vi "Save File DOE Create Filename Sub.vi"(8 "Error In":errorcluster, 9 "Filepath":T1, 10 "LV Program":T9=enum."DOE Stand", 11 "Appliance Details":T3={"FileVersionInfo"={"FileVersion"="", "ProductName"="", "InternalName"="", "CompanyName"="", "LegalCopyright"="", "FileDescription"=""}, "Dishwasher Info"={"Open Cup Weight (gm):"=0.0, "Auto Cup Weight (gm):"=0.0, "Detergent-Dish:"="", "Inlet Temperature-Dish:"="", "Cycle Mode-Dish:"="", "Unit Control-Dish:"="", "Manufacturer-Dish:"=""}, "Washer Info"={"Hot Water Temperature (Fahrenheit):"="", "Cold Water Temperature (Fahrenheit):"="", "Capacity (cu.ft):"=0.0, "Initial Cloth Weight:"=0.0, "Cloth Lot:"=0, "Model Family:"="", "Program Name:"="", "Cycle Selection:"="", "Wash Temperature:"="", "Rinse Temperature:"="", "Load Size:"=""}, "File Name Output Array"=[], "Calibration Output Array"=[], "Appliance Common"={"Engineer:"="", "Model Number:"="", "Serial Number:"="", "Comments:"="", "Station ID:"="", "Technician:"="", "TR Number:"="", "Lab ID:"="", "Voltage:"="", "Water Pressure (PSI):"="", "Test Date:"="", "Computer Name:"="", "IP Address:"="", "Ambient RH:"="", "Frequency:"="", "Build:"="", "Filename:"="", "Test Type:"="", "Load Run #:"=0, "Ambient Temperature (F):"="", "File Path:"=path "", "Cycles Per Year"=60}, "Water Heater"={"Heating Mode:"=""}, "Dryer"={"Heat Setting:"="", "Washer Water Temperature (60 ± 5°F):"=60, "Water Hardness (PPM):"=17, "Dryness Setting:"="", "Dryer Type:"="", "Exhaust:"="", "Drying Cycle:"="", "Load Type:"="", "Nominal Load Weight"="", "Dryer Initial IMC Data"={"Measured IMC (lbs)"=7.0, "Actual Initial RMC (%)"=7.0, "RMC (Desired %)"=100.0, "Bone Dry Wt(lbs)"=7.0, "Tolerance(%)"=5.0, "Actual Final RMC (%)"=7.0, "CEF (lbf/kWh)"=0.0, "Minimum Weight (lbf)"=0.0, "Average Weight (lbf)"=0.0, "Maximum Weight (lbf)"=0.0, "Measured IMC In Range?"=FALSE, "Moisture Reduction Factor"=55.5, "Field Use Factor"=1.04, "Empty Dryer Cold Weigth"=0.0, "Energy Standard"=enum."D2-Automatic Dryer", "Weight Cloth (lbs)"=0.0, "Relative Moisture Content (%)"=0.0, "Relative Moisture Content - Avg (%)"=0.0}}} {"Dryer"."Dryer Initial IMC Data"."Maximum Weight (lbf)" format="%03_6g"; "Dryer"."Dryer Initial IMC Data"."Average Weight (lbf)" format="%03_6g"; "Dryer"."Dryer Initial IMC Data"."Minimum Weight (lbf)" format="%03_6g"; "Dryer"."Dryer Initial IMC Data"."CEF (lbf/kWh)" format="%03_6g"; "Dryer"."Dryer Initial IMC Data"."Actual Final RMC (%)" format="%03_6g"; "Dryer"."Dryer Initial IMC Data"."Tolerance(%)" format="%0#_6g"; "Dryer"."Dryer Initial IMC Data"."Bone Dry Wt(lbs)" format="%03_6g"; "Dryer"."Dryer Initial IMC Data"."RMC (Desired %)" format="%0#_6g"; "Dryer"."Dryer Initial IMC Data"."Actual Initial RMC (%)" format="%03_6g"; "Dryer"."Dryer Initial IMC Data"."Measured IMC (lbs)" format="%0#_6g"}) -> (0 "Error Out":errorcluster, 2 "Filepath Output":T1, 3 "Appliance Details Output":T3={"FileVersionInfo"={"FileVersion"="", "ProductName"="", "InternalName"="", "CompanyName"="", "LegalCopyright"="", "FileDescription"=""}, "Dishwasher Info"={"Open Cup Weight (gm):"=0.0, "Auto Cup Weight (gm):"=0.0, "Detergent-Dish:"="", "Inlet Temperature-Dish:"="", "Cycle Mode-Dish:"="", "Unit Control-Dish:"="", "Manufacturer-Dish:"=""}, "Washer Info"={"Hot Water Temperature (Fahrenheit):"="", "Cold Water Temperature (Fahrenheit):"="", "Capacity (cu.ft):"=0.0, "Initial Cloth Weight:"=0.0, "Cloth Lot:"=0, "Model Family:"="", "Program Name:"="", "Cycle Selection:"="", "Wash Temperature:"="", "Rinse Temperature:"="", "Load Size:"=""}, "File Name Output Array"=[], "Calibration Output Array"=[], "Appliance Common"={"Engineer:"="", "Model Number:"="", "Serial Number:"="", "Comments:"="", "Station ID:"="", "Technician:"="", "TR Number:"="", "Lab ID:"="", "Voltage:"="", "Water Pressure (PSI):"="", "Test Date:"="", "Computer Name:"="", "IP Address:"="", "Ambient RH:"="", "Frequency:"="", "Build:"="", "Filename:"="", "Test Type:"="", "Load Run #:"=0, "Ambient Temperature (F):"="", "File Path:"=path "", "Cycles Per Year"=60}, "Water Heater"={"Heating Mode:"=""}, "Dryer"={"Heat Setting:"="", "Washer Water Temperature (60 ± 5°F):"=60, "Water Hardness (PPM):"=17, "Dryness Setting:"="", "Dryer Type:"="", "Exhaust:"="", "Drying Cycle:"="", "Load Type:"="", "Nominal Load Weight"="", "Dryer Initial IMC Data"={"Measured IMC (lbs)"=7.0, "Actual Initial RMC (%)"=7.0, "RMC (Desired %)"=100.0, "Bone Dry Wt(lbs)"=7.0, "Tolerance(%)"=5.0, "Actual Final RMC (%)"=7.0, "CEF (lbf/kWh)"=0.0, "Minimum Weight (lbf)"=0.0, "Average Weight (lbf)"=0.0, "Maximum Weight (lbf)"=0.0, "Measured IMC In Range?"=FALSE, "Moisture Reduction Factor"=55.5, "Field Use Factor"=1.04, "Empty Dryer Cold Weigth"=0.0, "Energy Standard"=enum."D2-Automatic Dryer", "Weight Cloth (lbs)"=0.0, "Relative Moisture Content (%)"=0.0, "Relative Moisture Content - Avg (%)"=0.0}}} {"Dryer"."Dryer Initial IMC Data"."Maximum Weight (lbf)" format="%03_6g"; "Dryer"."Dryer Initial IMC Data"."Average Weight (lbf)" format="%03_6g"; "Dryer"."Dryer Initial IMC Data"."Minimum Weight (lbf)" format="%03_6g"; "Dryer"."Dryer Initial IMC Data"."CEF (lbf/kWh)" format="%03_6g"; "Dryer"."Dryer Initial IMC Data"."Actual Final RMC (%)" format="%03_6g"; "Dryer"."Dryer Initial IMC Data"."Tolerance(%)" format="%0#_6g"; "Dryer"."Dryer Initial IMC Data"."Bone Dry Wt(lbs)" format="%03_6g"; "Dryer"."Dryer Initial IMC Data"."RMC (Desired %)" format="%0#_6g"; "Dryer"."Dryer Initial IMC Data"."Actual Initial RMC (%)" format="%03_6g"; "Dryer"."Dryer Initial IMC Data"."Measured IMC (lbs)" format="%0#_6g"})   [LabVIEW 2016, in "File Setup.lvlib"]
uses:
  File Setup.lvlib
  Save File.lvlib
  File Setup (Public)/Type Definition/Save File DOE LabView Program.ctl
  File Setup (Public)/Type Definition/Save File DISH Dishwasher Details.ctl
  <vilib>/Platform/fileVersionInfo.llb/FileVersionInformation.ctl
  File Setup (Public)/Type Definition/Save File DOE Data Save Filepaths.ctl
  File Setup (Public)/Type Definition/Save File DOE File Path Control.ctl
  Custom Pallet Controls/Custom Pallet String.ctl
  File Setup (Public)/Type Definition/DPT IMC Data.ctl
  Washer DOE/Type Definitions/DOE Appliance Common.ctl
  Washer DOE/Type Definitions/DOE Dryer Standard.ctl
panel:
  in  "File Extension:":string="csv"
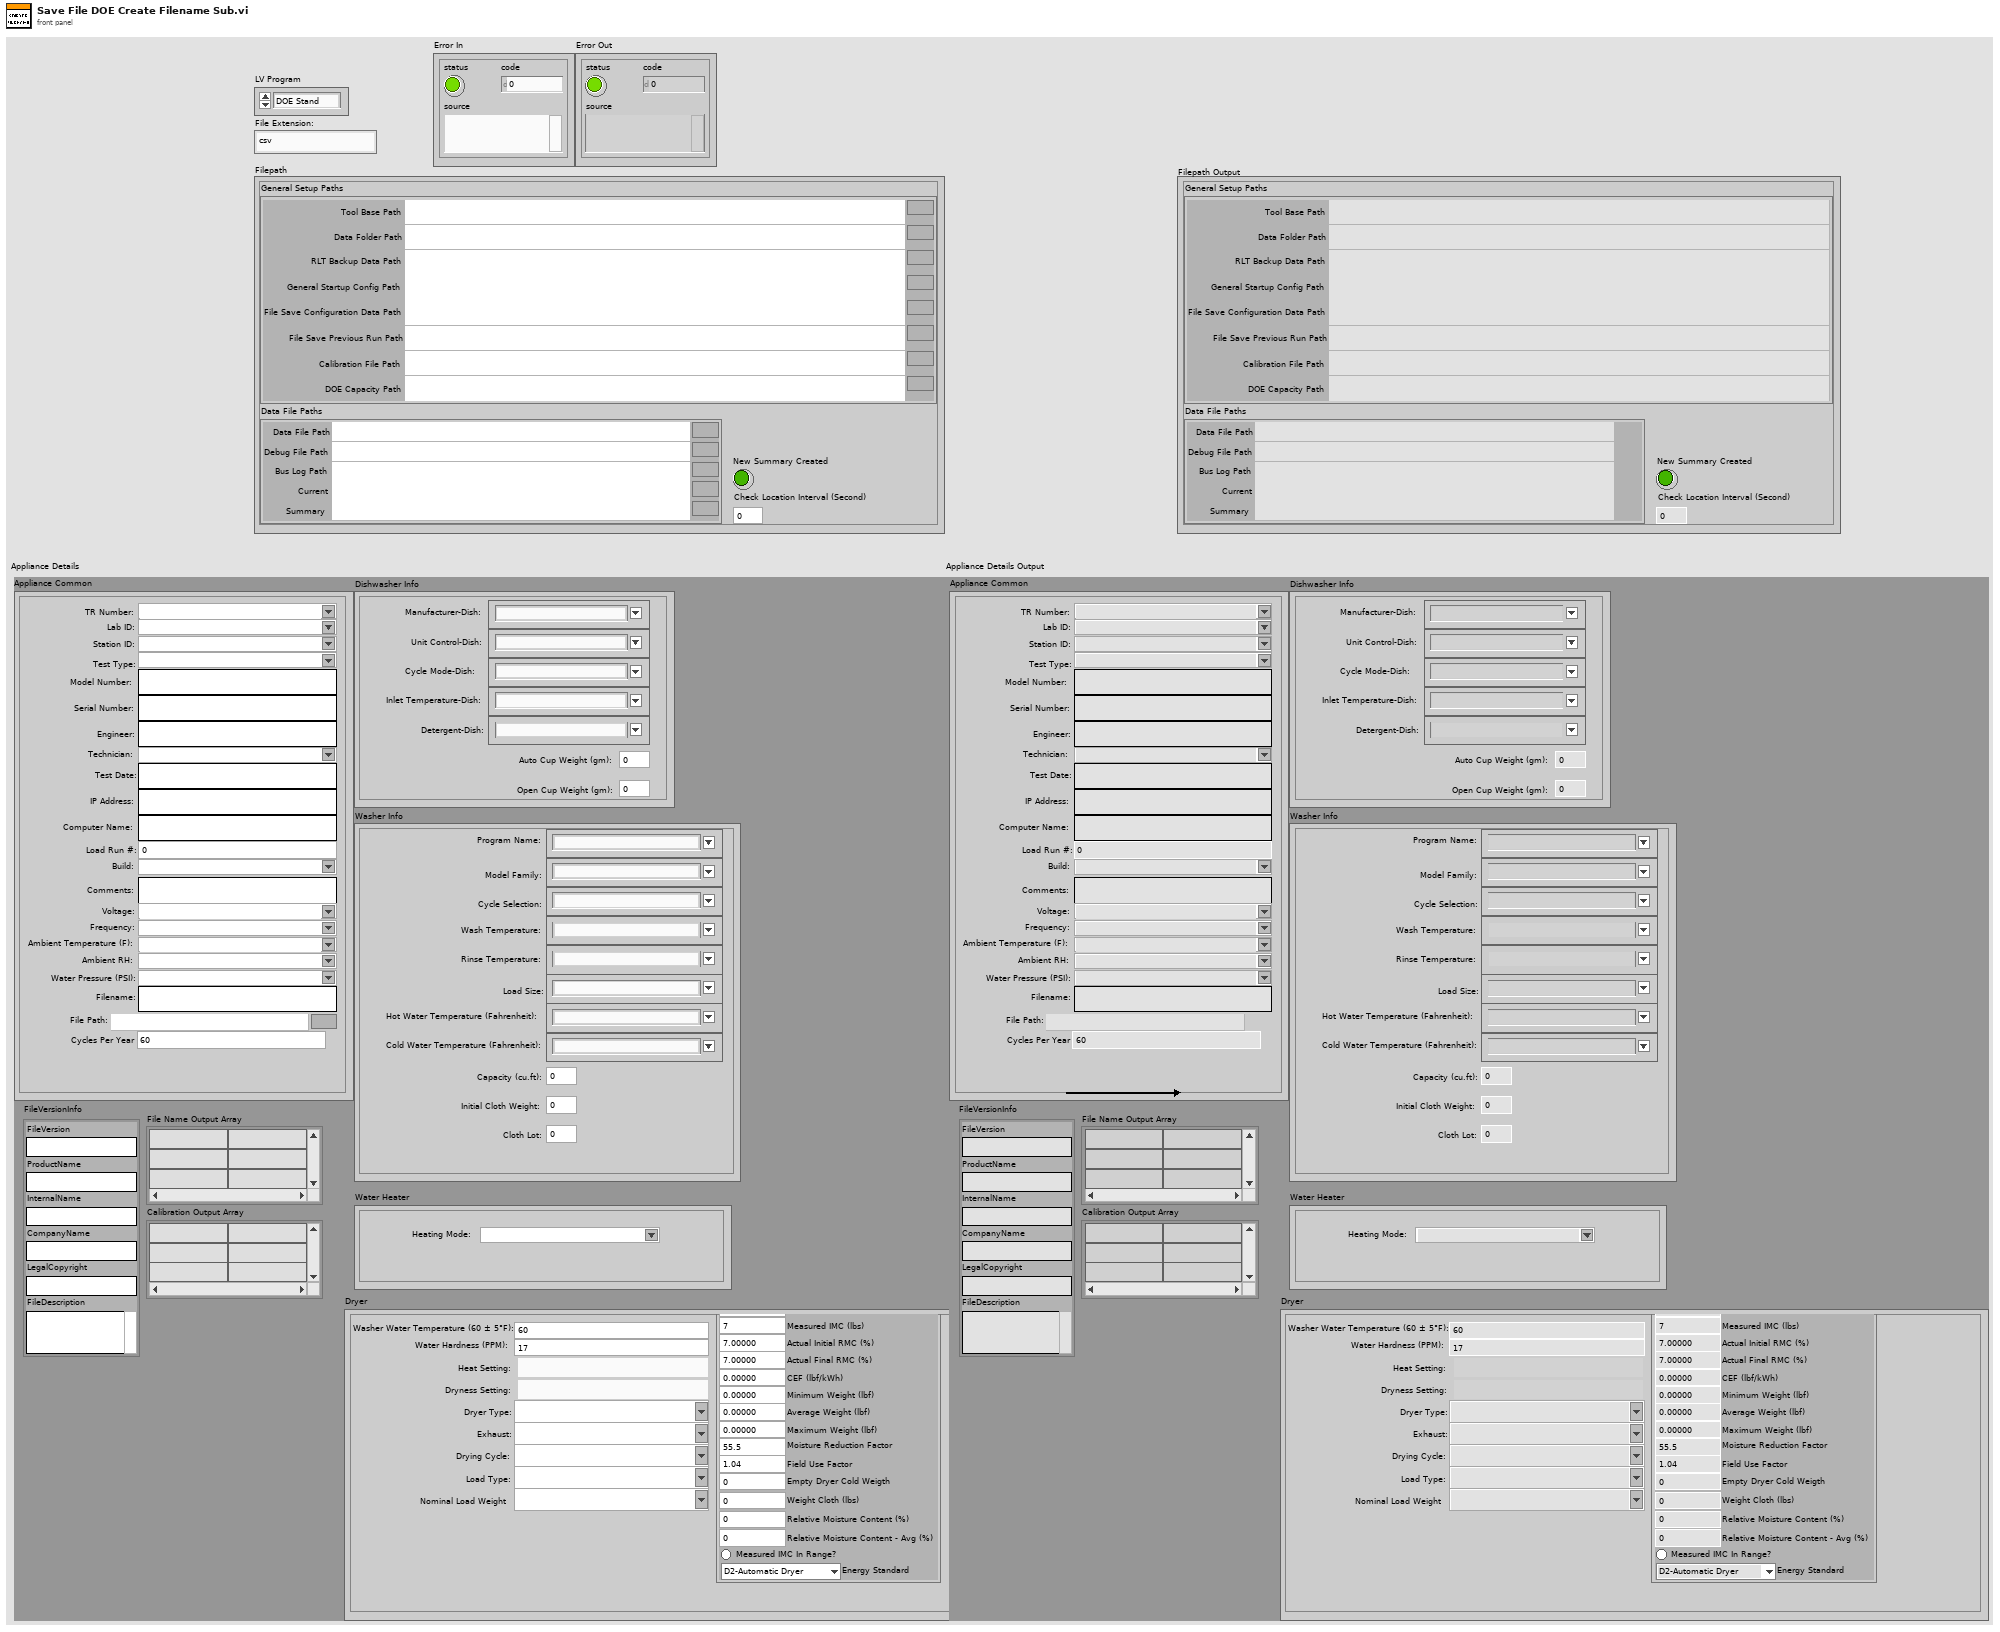
[diagram p1: front panel]
types:
  T1 = typedef "File Setup.lvlib/Save File DOE File Path Control.ctl" = cluster{"General Setup Paths":cluster{"Calibration File Path":path, "DOE Capacity Path":path, "Data Folder Path":path, "RLT Backup Data Path":path, "Tool Base Path":path, "General Startup Config Path":path, "File Save Previous Run Path":path, "File Save Configuration Data Path":path}, "Data File Paths":T2, "New Summary Created":bool, "Check Location Interval (Second)":i32}
  T2 = typedef "File Setup.lvlib/Save File DOE Data Save Filepaths.ctl" = cluster{"Data File Path":path, "Debug File Path":path, "Bus Log Path":path, "Current":path, "Summary":path}
  T3 = typedef "File Setup.lvlib/Save File DISH Dishwasher Details.ctl" = cluster{"FileVersionInfo":T4, "Dishwasher Info":cluster{"Open Cup Weight (gm):":dbl, "Auto Cup Weight (gm):":dbl, "Detergent-Dish:":string, "Inlet Temperature-Dish:":string, "Cycle Mode-Dish:":string, "Unit Control-Dish:":string, "Manufacturer-Dish:":string}, "Washer Info":cluster{"Hot Water Temperature (Fahrenheit):":string, "Cold Water Temperature (Fahrenheit):":string, "Capacity (cu.ft):":dbl, "Initial Cloth Weight:":dbl, "Cloth Lot:":i32, "Model Family:":string, "Program Name:":string, "Cycle Selection:":string, "Wash Temperature:":string, "Rinse Temperature:":string, "Load Size:":string}, "File Name Output Array":string[][], "Calibration Output Array":string[][], "Appliance Common":T5, "Water Heater":cluster{"Heating Mode:":string}, "Dryer":cluster{"Heat Setting:":T6, "Washer Water Temperature (60 ± 5°F):":u16, "Water Hardness (PPM):":u16, "Dryness Setting:":T6, "Dryer Type:":string, "Exhaust:":string, "Drying Cycle:":string, "Load Type:":string, "Nominal Load Weight":string, "Dryer Initial IMC Data":T7}}
  T4 = typedef "FileVersionInformation.ctl" = cluster{"FileVersion":string, "ProductName":string, "InternalName":string, "CompanyName":string, "LegalCopyright":string, "FileDescription":string}
  T5 = typedef "DOE Appliance Common.ctl" = cluster{"Engineer:":string, "Model Number:":string, "Serial Number:":string, "Comments:":string, "Station ID:":string, "Technician:":string, "TR Number:":string, "Lab ID:":string, "Voltage:":string, "Water Pressure (PSI):":string, "Test Date:":string, "Computer Name:":string, "IP Address:":string, "Ambient RH:":string, "Frequency:":string, "Build:":string, "Filename:":string, "Test Type:":string, "Load Run #:":i32, "Ambient Temperature (F):":string, "File Path:":path, "Cycles Per Year":u32}
  T6 = typedef "Custom Pallet String.ctl" = string
  T7 = typedef "DPT IMC Data.ctl" = cluster{"Measured IMC (lbs)":dbl, "Actual Initial RMC (%)":dbl, "RMC (Desired %)":dbl, "Bone Dry Wt(lbs)":dbl, "Tolerance(%)":dbl, "Actual Final RMC (%)":dbl, "CEF (lbf/kWh)":dbl, "Minimum Weight (lbf)":dbl, "Average Weight (lbf)":dbl, "Maximum Weight (lbf)":dbl, "Measured IMC In Range?":bool, "Moisture Reduction Factor":dbl, "Field Use Factor":dbl, "Empty Dryer Cold Weigth":dbl, "Energy Standard":T8, "Weight Cloth (lbs)":dbl, "Relative Moisture Content (%)":dbl, "Relative Moisture Content - Avg (%)":dbl}
  T8 = typedef "DOE Dryer Standard.ctl" = enum16{"D2-Automatic Dryer", "D2-Timer Dryer", "D1-Automatic Dryer", "D1-Timer Dryer", "Other"}
  T9 = typedef "File Setup.lvlib/Save File DOE LabView Program.ctl" = enum16{"No Name Found", "DOE Stand", "Dishwasher Kitchen", "Portable Stand", "HEWH", "Dryer", "Dryer WILT", "HCC", "PRAT", "HEWH RLT"}
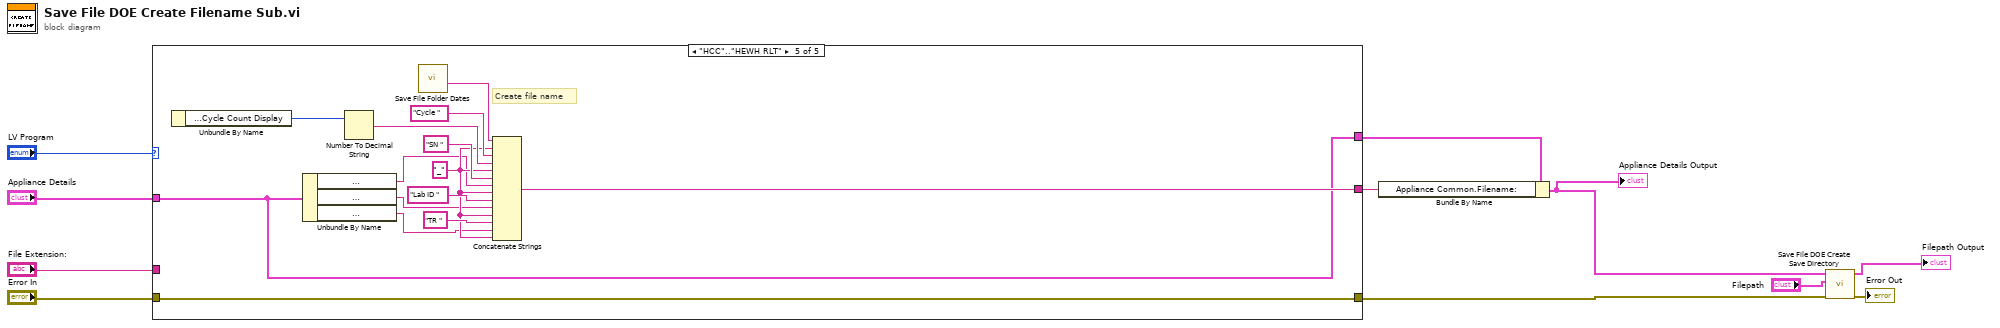
[diagram p0: block diagram]
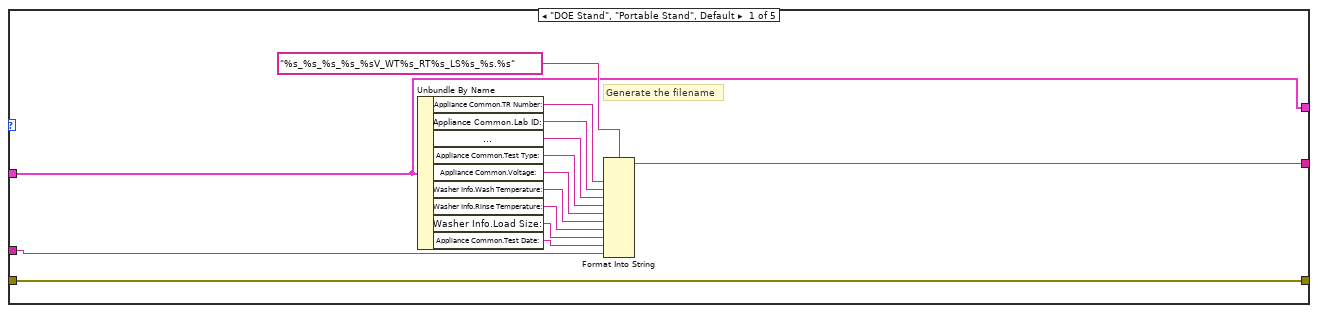
[diagram p2: hidden frame]
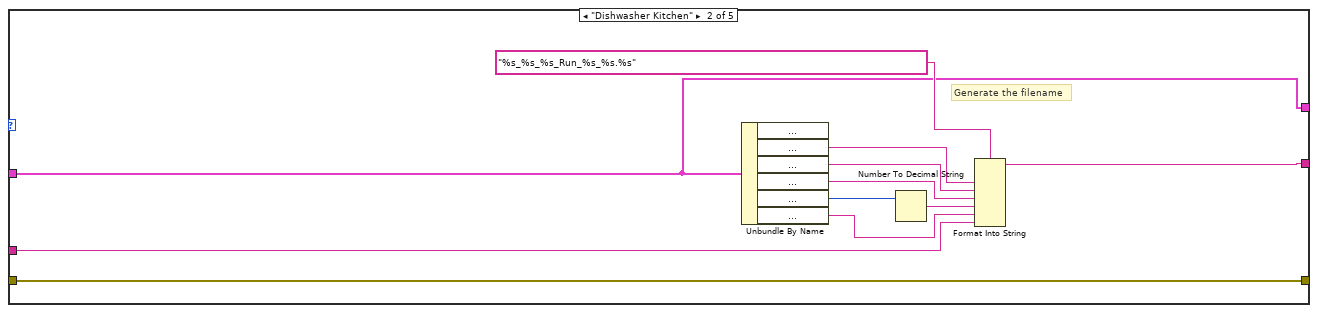
[diagram p3: hidden frame]
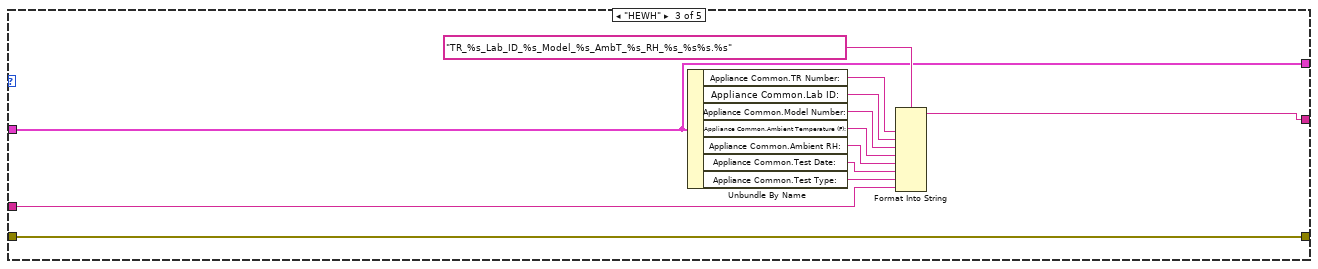
[diagram p4: hidden frame]
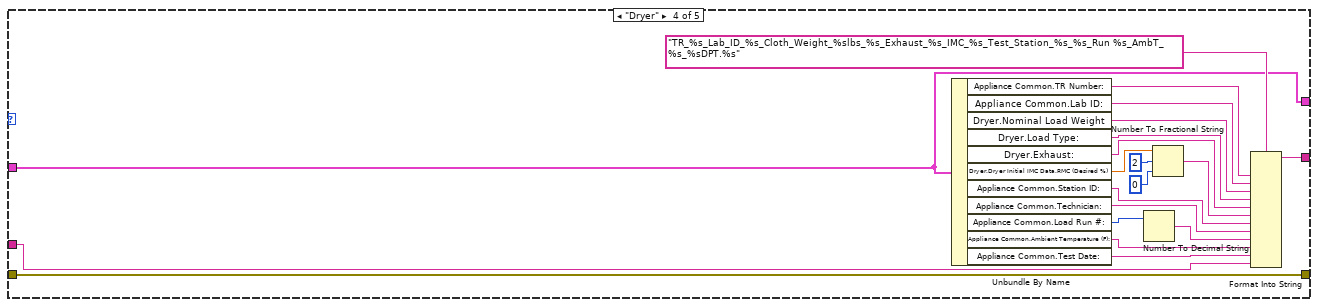
[diagram p5: hidden frame]
diagram:
  n1 = case shown="\"HCC\"..\"HEWH RLT\"" "LV Program" {
    tunnel: [w25 w33 w41 w50 w74] -> w8
    tunnel: "File Extension:" -> [w15 w30 w42 w67 _]
    tunnel: "Appliance Details" -> [w13 w27 w38 w51 w70]
    tunnel: [w13 w27 w38 w51 w70] -> w7
    tunnel: "Error In" -> [w12 w26 w37 w49 w69]
    tunnel: [w12 w26 w37 w49 w69] -> w3
    frame "DOE Stand", "Portable Stand", Default {
      # "Generate the filename"
      n2 = Unbundle By Name(w13) -> ("Appliance Common.TR Number:"=w24:string, "Appliance Common.Lab ID:"=w23:string, "Appliance Common.Model Number:"=w21:string, "Appliance Common.Test Type:"=w14:string, "Appliance Common.Voltage:"=w22:string, "Washer Info.Wash Temperature:"=w19:string, "Washer Info.Rinse Temperature:"=w18:string, "Washer Info.Load Size:"=w17:string, "Appliance Common.Test Date:"=w16:string)
      n3 = Format Into String(format string="%s_%s_%s_%s_%sV_WT%s_RT%s_LS%s_%s.%s", w24, w23, w21, w14, w22, w19, w18, w17, w16, w15) -> (resulting string=w25:string)  [unwired: 2 in, 1 out]
    }
    frame "Dishwasher Kitchen" {
      # "Generate the filename"
      n4 = Unbundle By Name(w27) -> ("Appliance Common.Lab ID:"=w34:string, "Appliance Common.Test Type:"=w35:string, "Appliance Common.Comments:"=w36:string, "Appliance Common.Load Run #:"=w29:i32, "Appliance Common.Test Date:"=w31:string)  [unwired: 1 out]
      n5 = Number To Decimal String(number=w29) -> (decimal integer string=w28:string)  [unwired: 1 in]
      n6 = Format Into String(format string="%s_%s_%s_Run_%s_%s.%s", w34, w35, w36, w28, w31, w30) -> (resulting string=w33:string)  [unwired: 2 in, 1 out]
    }
    frame "HEWH" {
      n7 = Unbundle By Name(w38) -> ("Appliance Common.TR Number:"=w40:string, "Appliance Common.Lab ID:"=w39:string, "Appliance Common.Model Number:"=w47:string, "Appliance Common.Ambient Temperature (F):"=w46:string, "Appliance Common.Ambient RH:"=w45:string, "Appliance Common.Test Date:"=w44:string, "Appliance Common.Test Type:"=w43:string)
      n8 = Format Into String(format string="TR_%s_Lab_ID_%s_Model_%s_AmbT_%s_RH_%s_%s%s.%s", w40, w39, w47, w46, w45, w44, w43, w42) -> (resulting string=w41:string)  [unwired: 2 in, 1 out]
    }
    frame "Dryer" {
      n9 = Unbundle By Name(w51) -> ("Appliance Common.TR Number:"=w52:string, "Appliance Common.Lab ID:"=w53:string, "Dryer.Nominal Load Weight"=w54:string, "Dryer.Load Type:"=w55:string, "Dryer.Exhaust:"=w56:string, "Dryer.Dryer Initial IMC Data.RMC (Desired %)"=w58:dbl, "Appliance Common.Station ID:"=w61:string, "Appliance Common.Technician:"=w62:string, "Appliance Common.Load Run #:"=w65:i32, "Appliance Common.Ambient Temperature (F):"=w64:string, "Appliance Common.Test Date:"=w66:string)
      n10 = Number To Decimal String(number=w65) -> (decimal integer string=w63:string)  [unwired: 1 in]
      n11 = Number To Fractional String(number=w58, width (-)=i16 2, precision (6)=i16 0) -> (F-format string=w57:string)  [unwired: 1 in]
      n12 = Format Into String(format string="TR_%s_Lab_ID_%s_Cloth_Weight_%slbs_%s_Exhaust_%s_IMC_%s_Test_Station_%s_%s_Run %s_AmbT_%s_%sDPT.%s", w52, w53, w54, w55, w56, w57, w61, w62, w63, w64, w66, w67) -> (resulting string=w50:string)  [unwired: 2 in, 1 out]
    }
    frame "HCC".."HEWH RLT" {
      w76 = "_" ("string")
      # "Create file name"
      n13 = Unbundle By Name() -> ("Display Data (RLT).Cycle Count Display"=w75:i32)  [unwired: 1 in]
      n14 = Unbundle By Name(w70) -> ("Appliance Common.Serial Number:"=w71:string, "Appliance Common.Lab ID:"=w72:string, "Appliance Common.TR Number:"=w73:string)
      n15 = Number To Decimal String(number=w75) -> (decimal integer string=w80:string)  [unwired: 1 in]
      n16 = call "Save File Folder Dates.vi"() -> ("Year/Month/Day"=w82:string)  [unwired: 8 in, 3 out]
      n17 = Concatenate Strings(w82, w76, "Cycle " ("string"), w80, w76, "SN " ("string"), w71, w76, "Lab ID " ("string"), w72, w76, "TR " ("string"), w73, w76) -> (w74:string)
    }
  }
  n18 = Bundle By Name(cluster=w7, "Appliance Common.Filename:"=w8) -> (w1:T3)
  "Appliance Details Output" <- w1
  n19 = call "Save File DOE Create Save Directory.vi"("error in (no error)"=w3, "Filepath"="Filepath", "Appliance Details Output"=w1) -> ("error out"=→"Error Out":errorcluster, "Filepath Output"=→"Filepath Output":T1)  [unwired: 7 in]
